vi "VLC-IP_File_Inizialize.vi"(8 "error in":errorcluster, 11 "FramePerSec":i32) -> (0 "error out":errorcluster, 1 "SamplingTime":i32, 2 "TemporaryFilePath":path)   [LabVIEW 2016]
uses:
  <vilib>/Utility/sysdir.llb/System Directory Type.ctl
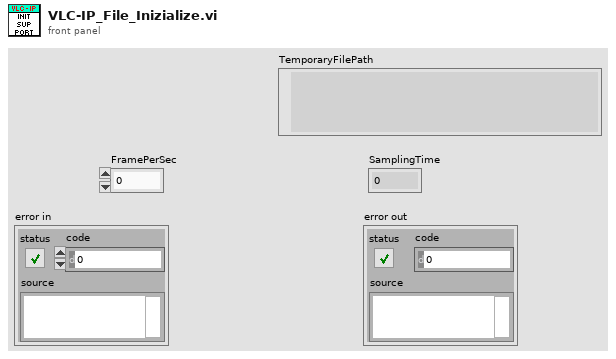
[diagram p1: front panel]
types:
  T1 = enum16{"open", "replace", "create", "open or create", "replace or create", "replace or create with confirmation"}
  T2 = typedef "System Directory Type.ctl" = i32
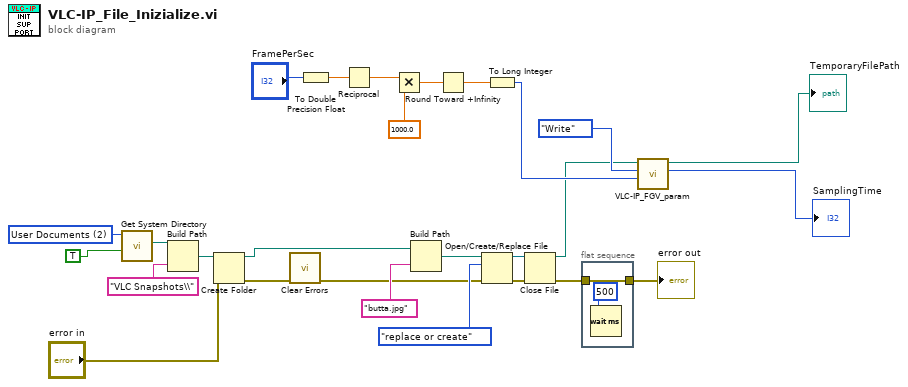
[diagram p0: block diagram]
diagram:
  w16 = T2 2 items=["User Home"=0, "User Desktop"=1, "User Documents"=2, "User Application Data"=3, "User Preferences"=4, "User Temporary"=5, "Public Documents"=6, "Public Application Data"=7, "Public Preferences"=8, "Public Cache"=13, "System Core Libraries"=9, "System Installed Libraries"=10, "Application Files"=11, "Boot Volume Root"=12] ("system directory type")
  n1 = call <vilib>:"Get System Directory.vi"("create directory if not found? (F)"=TRUE, "system directory type"=w16) -> ("system directory"=w17:path)  [unwired: 9 in]
  n2 = Build Path(base path=w17, name or relative path="VLC Snapshots\\") -> (appended path=w19:path)
  n3 = Create Folder(path (use dialog)=w19, error in="error in") -> (created path=w21:path, error out=w22:errorcluster)  [unwired: 1 in, 1 out]
  n4 = call <vilib>:"Clear Errors.vi"("error in (no error)"=w22) -> ("error out"=w9:errorcluster)  [unwired: 5 in, 1 out]
  n5 = To Double Precision Float(number="FramePerSec") -> (double precision float=w14:dbl)
  n6 = Reciprocal(x=w14) -> (1/x=w13:dbl)
  n7 = Multiply(x=w13, y=1000.0) -> (x*y=w8:dbl)
  n8 = Build Path(base path=w21, name or relative path="butta.jpg") -> (appended path=w3:path)
  n9 = Round Toward +Infinity(x=w8) -> (ceil(x): smallest int >= x=w12:dbl)
  n10 = Open/Create/Replace File(file path (use dialog)=w3, error in=w9, operation (0:open)=T1."replace or create") -> (refnum out=w25:refnum<file>, error out=w24:errorcluster)  [unwired: 3 in, 1 out]
  n11 = To Long Integer(number=w12) -> (32bit integer=w5:i32)
  n12 = Close File(refnum=w25, error in=w24) -> (path=w1:path, error out=w26:errorcluster)
  n13 = flat-sequence {
    tunnel: w26 -> [w29]
    tunnel: [w29] -> w27
    frame #0 {
      n14 = Wait (ms)(milliseconds to wait=u32 500) -> ()  [unwired: 1 out]
    }
  }
  n15 = call "VLC-IP_FGV_param.vi"("SamplingTime_in"=w5, "Mode"=enum16{"Read", "Write"}."Write", "TemporaryFilePath_in"=w1) -> ("SamplingTime_out"=→"SamplingTime":i32, "TemporaryFilePath_out"=→"TemporaryFilePath":path)  [unwired: 7 in]
  "error out" <- w27
